vi "sub_rplidar_init-recovery.vi"() -> (0 "error out":errorcluster caption="에러 출력")   [LabVIEW 2019]
uses:
  Ctrl/rplidar_cmd.ctl
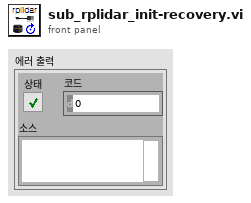
[diagram p1: front panel]
types:
  T1 = typedef "rplidar_cmd.ctl" = enum16{"init", "health", "spin", "scan", "read", "stop", "close"}
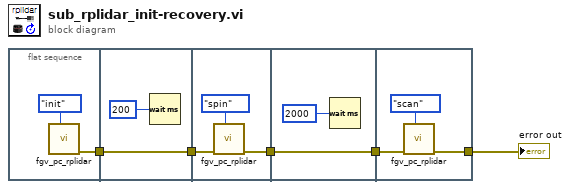
[diagram p0: block diagram]
diagram:
  n1 = flat-sequence {
    tunnel: [w7] -> w5
    tunnel: w5 -> [w9]
    tunnel: [w9] -> w4
    tunnel: w4 -> [w11]
    tunnel: [w10] -> w3
    tunnel: w3 -> [w14]
    tunnel: [w14] -> w2
    tunnel: w2 -> [w16]
    tunnel: [w15] -> w1
    frame #0 {
      n2 = call "fgv_pc_rplidar.vi"("cmd"=rplidar_cmd."init") -> ("error out"=w7:errorcluster)  [unwired: 8 in, 2 out]
    }
    frame #1 {
      n3 = Wait (ms)(milliseconds to wait=u32 200) -> ()  [unwired: 1 out]
    }
    frame #2 {
      n4 = call "fgv_pc_rplidar.vi"("cmd"=rplidar_cmd."spin", "error in"=w11) -> ("error out"=w10:errorcluster)  [unwired: 7 in, 2 out]
    }
    frame #3 {
      n5 = Wait (ms)(milliseconds to wait=u32 2000) -> ()  [unwired: 1 out]
    }
    frame #4 {
      n6 = call "fgv_pc_rplidar.vi"("cmd"=rplidar_cmd."scan", "error in"=w16) -> ("error out"=w15:errorcluster)  [unwired: 7 in, 2 out]
    }
  }
  "error out" <- w1
